vi "user input.vi"(8 "error in":errorcluster, 11 "Session":refnum<k21>) -> (0 "error out":errorcluster, 3 "Inputs from system":T1)   [LabVIEW 2014, in "RTResourceUtilitzation runtime.lvclass"]
uses:
  RTResourceUtilitzation runtime.lvclass
  input user data.ctl
  <vilib>/Analysis/baseanly.llb/Mean (DBL).vi
  <resource>/objmgr/nisysapi.rc
  <vilib>/NI_Real-Time Target Support.lvlib
  <vilib>/Analysis/NI_AALBase.lvlib
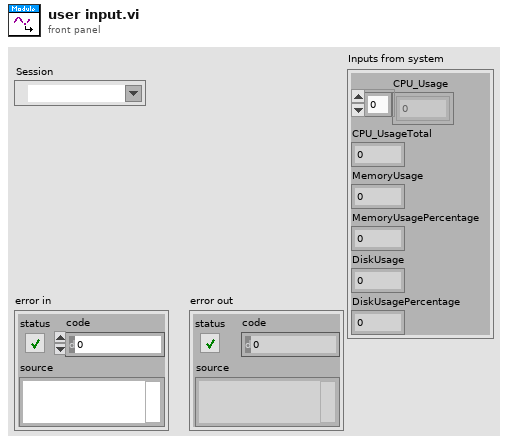
[diagram p1: front panel]
types:
  T1 = typedef "RTResourceUtilitzation runtime.lvclass/input user data.ctl" = cluster{"CPU_Usage":dbl[], "CPU_UsageTotal":dbl, "MemoryUsage":dbl, "MemoryUsagePercentage":dbl, "DiskUsage":dbl, "DiskUsagePercentage":dbl}
  T2 = typedef "NI_Real-Time Target Support.lvlib/RT CPU Load.ctl" = cluster{"Total (%)":dbl, "Time Critical (%)":dbl, "Timed Structures (%)":dbl, "High (%)":dbl, "Above Normal (%)":dbl, "Normal (%)":dbl, "Background (%)":dbl, "Idle (%)":dbl, "ISR (%)":dbl}
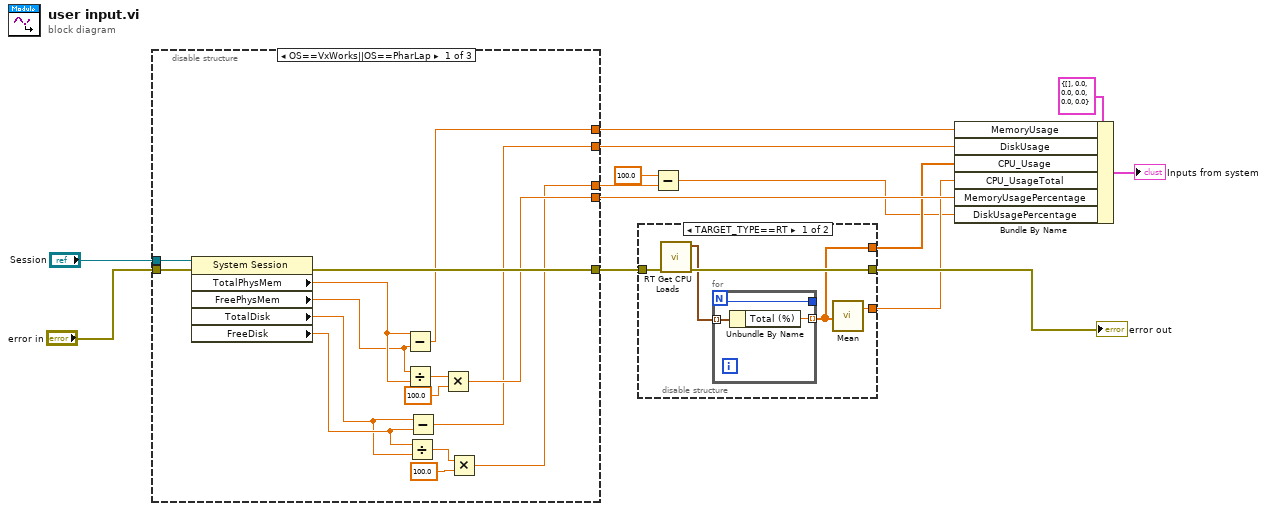
[diagram p0: block diagram]
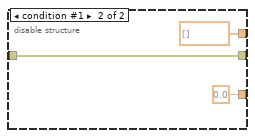
[diagram p2: hidden frame]
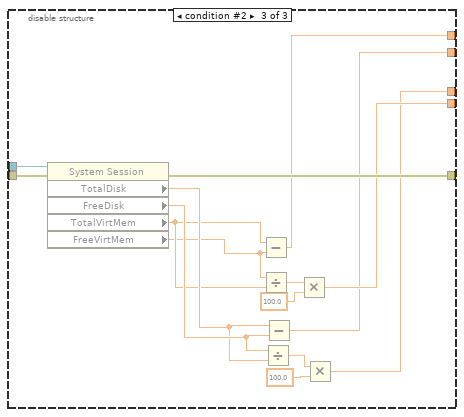
[diagram p4: hidden frame]
diagram:
  n1 = disable-structure shown="OS==VxWorks||OS==PharLap" {
    disable-tunnel: "Session" -> [w29 _ w45]
    disable-tunnel: "error in" -> [w28 w30 w44]
    disable-tunnel: [w27 w30 w43] -> w7
    disable-tunnel: [w26 _ w42] -> w10
    disable-tunnel: [w24 _ w40] -> w9
    disable-tunnel: [w17 _ w33] -> w8
    disable-tunnel: [w18 _ w34] -> w3
    frame condition #0 (active) {
      n2 = property class="System Session"(reference=w29, error in=w28) -> (error out=w27:errorcluster, "TotalPhysMem"=w16:dbl, "FreePhysMem"=w15:dbl, "TotalDisk"=w19:dbl, "FreeDisk"=w20:dbl)  [unwired: 1 out]
      n3 = Subtract(x=w16, y=w15) -> (x-y=w26:dbl)
      n4 = Divide(x=w15, y=w16) -> (x/y=w25:dbl)
      n5 = Divide(x=w20, y=w19) -> (x/y=w21:dbl)
      n6 = Subtract(x=w19, y=w20) -> (x-y=w17:dbl)
      n7 = Multiply(x=w25, y=100.0) -> (x*y=w24:dbl)
      n8 = Multiply(x=w21, y=100.0) -> (x*y=w18:dbl)
    }
    frame condition #1 {
    }
    frame condition #2 {
      n9 = property class="System Session"(reference=w45, error in=w44) -> (error out=w43:errorcluster, "TotalDisk"=w35:dbl, "FreeDisk"=w36:dbl, "TotalVirtMem"=w32:dbl, "FreeVirtMem"=w31:dbl)  [unwired: 1 out]
      n10 = Subtract(x=w32, y=w31) -> (x-y=w42:dbl)
      n11 = Divide(x=w31, y=w32) -> (x/y=w41:dbl)
      n12 = Divide(x=w36, y=w35) -> (x/y=w37:dbl)
      n13 = Subtract(x=w35, y=w36) -> (x-y=w33:dbl)
      n14 = Multiply(x=w41, y=100.0) -> (x*y=w40:dbl)
      n15 = Multiply(x=w37, y=100.0) -> (x*y=w34:dbl)
    }
  }
  n16 = disable-structure shown="TARGET_TYPE==RT" {
    disable-tunnel: w7 -> [w50 w55]
    disable-tunnel: [w49 w55] -> w6
    disable-tunnel: [w47 0.0 ("mean")] -> w4
    disable-tunnel: [w46 dbl[] []] -> w5
    frame condition #0 (active) {
      n17 = call <vilib>:"RT Get CPU Loads.vi"("error in (no error)"=w50) -> ("error out"=w49:errorcluster, "CPU loads"=w48:T2[])  [unwired: 9 in]
      n18 = for {
        N -> [w51]
        tunnel: w48 -> [w53] mode=indexing
        tunnel: [w52] -> w46 mode=indexing
        tunnel: [w51] -> _
        n19 = Unbundle By Name(w53) -> ("Total (%)"=w52:dbl)
      }
      n20 = call-poly <vilib>:"Mean.vi"("X"=w46) -> ("mean"=w47:dbl)  [unwired: 1 out]
    }
    frame condition #1 {
    }
  }
  "error out" <- w6
  n21 = Subtract(x=100.0, y=w3) -> (x-y=w1:dbl)
  n22 = Bundle By Name(cluster=T1 {"CPU_Usage"=[], "CPU_UsageTotal"=0.0, "MemoryUsage"=0.0, "MemoryUsagePercentage"=0.0, "DiskUsage"=0.0, "DiskUsagePercentage"=0.0} ("Inputs from system"), "MemoryUsage"=w10, "DiskUsage"=w8, "CPU_Usage"=w5, "CPU_UsageTotal"=w4, "MemoryUsagePercentage"=w9, "DiskUsagePercentage"=w1) -> (→"Inputs from system":T1)
